vi "Windows.UpdateTime.vi"(8 "error in (no error)":errorcluster, 11 "cmdtime path":path) -> (0 "error out":errorcluster, 2 "cmdtime info":string[](array[string]), 3 "level (Info)":T1=enum."Info")   [LabVIEW 2015]
doc: "Update windows local time with the network time servers\n- use 3rd party freeware application (cmdtime)\n- store its events to log them in application event logger\n\nAll hosts connected to Jahont Server should have the same local time for results comparison"
uses:
  EventLog/EventLog.EventLevel.ctl
panel:
  out "standard output":string
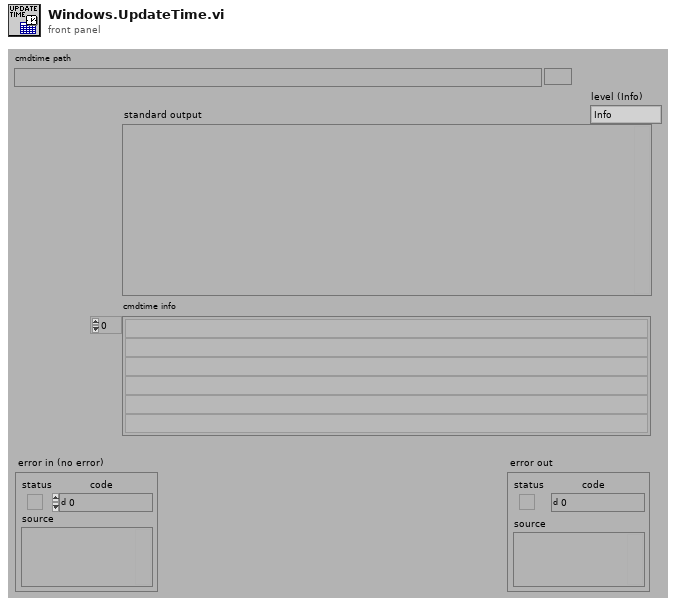
[diagram p1: front panel]
types:
  T1 = typedef "EventLog.EventLevel.ctl" = enum8{"Debug", "Info", "Warning", "Error"}
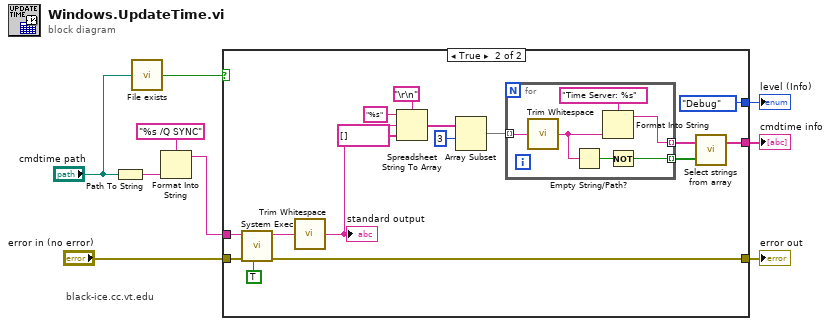
[diagram p0: block diagram]
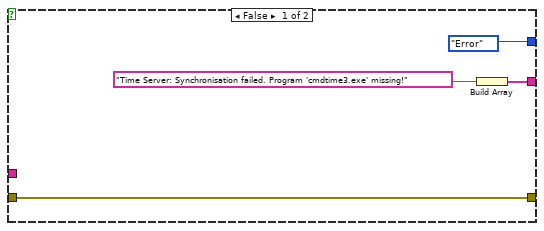
[diagram p2: hidden frame]
diagram:
  # "black-ice.cc.vt.edu"
  n1 = Path To String(path="cmdtime path") -> (string=w7:string)
  n2 = call "File exists.vi"("file path"="cmdtime path") -> ("exists?"=w2:bool)  [unwired: 4 in]
  n3 = Format Into String(format string="%s /Q SYNC", w7) -> (resulting string=w6:string)  [unwired: 2 in, 1 out]
  n4 = case shown="True" w2 {
    tunnel: "error in (no error)" -> [w10 w29]
    tunnel: [w10 w28] -> w8
    tunnel: w6 -> [_ w27]
    tunnel: [w12 w19] -> w4
    tunnel: [EventLog.EventLevel."Error" ("level (Info)") EventLog.EventLevel."Debug" ("level (Info)")] -> w1
    frame False {
      n5 = Build Array("Time Server: Synchronisation failed. Program 'cmdtime3.exe' missing!" ("explanation")) -> (w12:string[])
    }
    frame True {
      n6 = call <vilib>:"System Exec.vi"("run minimized? (F)"=TRUE, "error in (no error)"=w29, "command line"=w27) -> ("error out"=w28:errorcluster, "standard output"=w26:string)  [unwired: 5 in, 2 out]
      n7 = call <vilib>:"Trim Whitespace.vi"("string"=w26) -> ("trimmed string"=w22:string)  [unwired: 1 in]
      "standard output" <- w22
      n8 = Spreadsheet String To Array(delimiter (Tab)="\r\n", format string="%s", spreadsheet string=w22, array type (2D Dbl)=string[] []) -> (array=w18:string[])
      n9 = Array Subset(array=w18, index=3) -> (w16:string[])  [unwired: 1 in]
      n10 = for {
        tunnel: w16 -> [w35] mode=indexing
        tunnel: [w33] -> w21 mode=indexing
        tunnel: [w30] -> w20 mode=indexing
        n11 = call <vilib>:"Trim Whitespace.vi"("string"=w35) -> ("trimmed string"=w32:string)  [unwired: 1 in]
        n12 = Empty String/Path?(string/path=w32) -> (empty?=w34:bool)
        n13 = Format Into String(format string="Time Server: %s", w32) -> (resulting string=w30:string)  [unwired: 2 in, 1 out]
        n14 = Not(x=w34) -> (.not. x?=w33:bool)
      }
      n15 = call "Select strings from array.vi"("selection array"=w21, "strings"=w20) -> ("selected strings"=w19:string[])  [unwired: 1 in]
    }
  }
  "error out" <- w8
  "cmdtime info" <- w4
  "level (Info)" <- w1
